vi "Internet Version Check.vi"(8 "error in":errorcluster, 9 "Prompt If Newer Version Available":bool=TRUE, 10 "Version In":dbl format="%.2f", 11 "Version File Name":string="ljstreamud.txt") -> (0 "error out":errorcluster, 1 "Newer Version Online":bool, 2 "Value (float)":dbl format="%.6f")   [LabVIEW 2021]
panel:
  out "Content":string
  out "Header":string
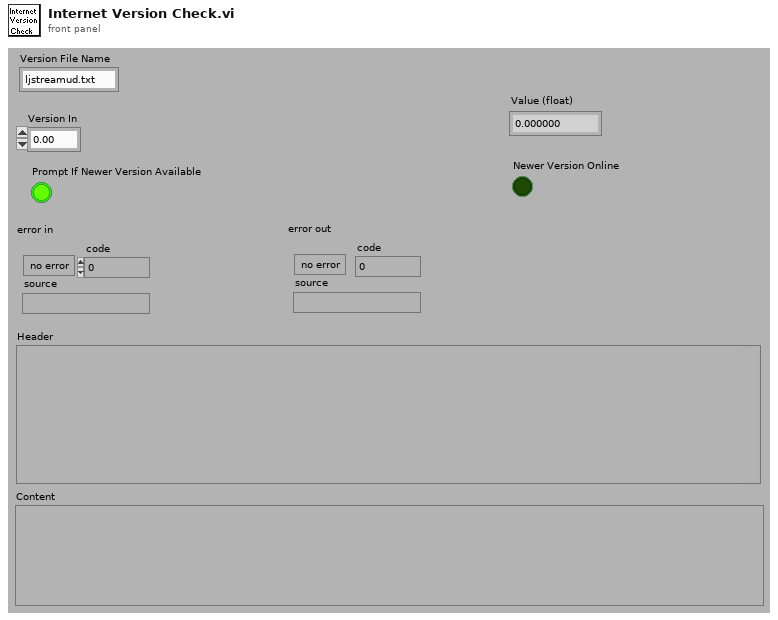
[diagram p1: front panel]
types:
  T1 = enum16{"Standard", "Buffered", "CRLF", "Immediate"}
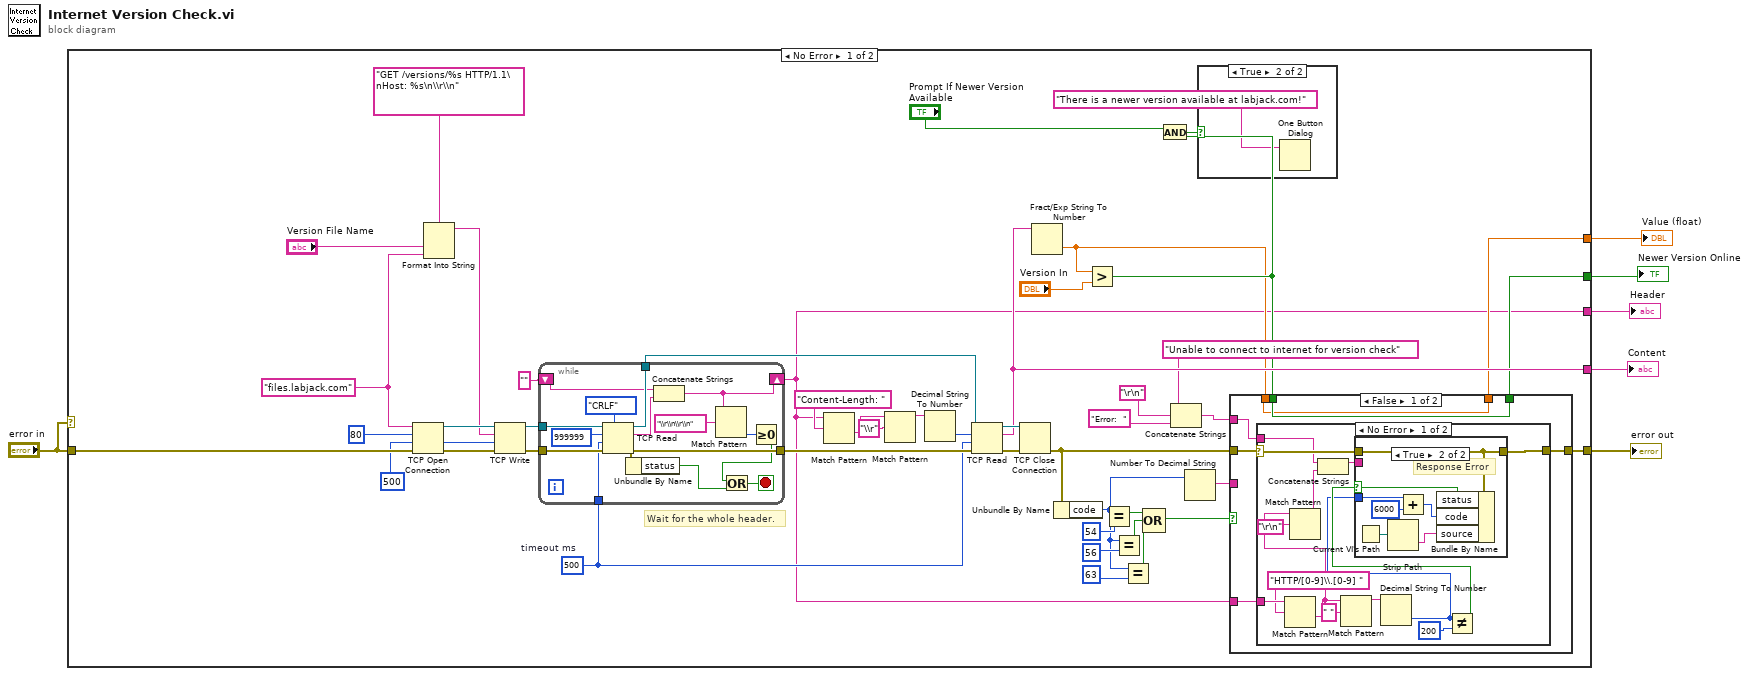
[diagram p0: block diagram]
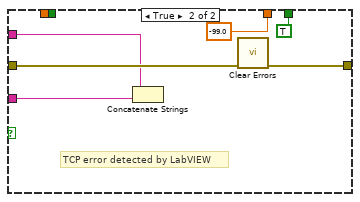
[diagram p4: hidden frame]
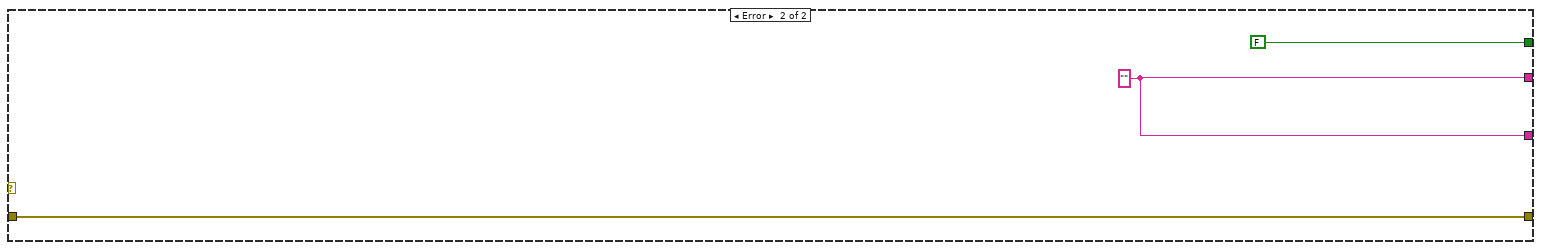
[diagram p6: hidden frame]
diagram:
  n1 = case shown="No Error" "error in" {
    tunnel: [w35 w106] -> w6
    tunnel: "error in" -> [w48 w106]
    tunnel: [w30 w105] -> w5
    tunnel: [w7 w105] -> w4
    tunnel: [w25 FALSE] -> w2
    tunnel: [w23 _] -> w1
    frame No Error {
      w22 = 500 ("timeout ms (60000)")
      w39 = 500  # timeout ms
      w32 = "files.labjack.com"
      # "Wait for the whole header."
      n2 = TCP Open Connection(address=w32, remote port or service name=u16 80 ("remote port"), timeout ms (60000)=w22, error in (no error)=w48) -> (connection ID=w52:refnum<k5>, error out=w50:errorcluster)  [unwired: 1 in]
      n3 = Format Into String(format string="GET /versions/%s HTTP/1.1\nHost: %s\n\\r\\n" ("Format String"), "Version File Name", w32) -> (resulting string=w31:string)  [unwired: 2 in, 1 out]
      n4 = TCP Write(connection ID=w52, data in=w31, error in (no error)=w50, 9:w22) -> (connection ID out=w51:refnum<k5>, error out=w49:errorcluster)  [unwired: 1 out]
      n5 = while {
        tunnel: w39 -> [w88]
        shift-left: "" -> [w98]
        shift-right: [w94] -> w7
        tunnel: [w96] -> w41
        tunnel: w49 -> [w100]
        tunnel: [w101] -> w38
        tunnel: w51 -> [w102]
        stop <- w90 stop-if-true
        n6 = TCP Read(connection ID=w102, bytes to read=999999, error in (no error)=w100, 7:T1."CRLF" ("mode (standard)"), 9:w88) -> (connection ID out=w101:refnum<k5>, data out=w97:string, error out=w96:errorcluster)
        n7 = Unbundle By Name(w96) -> ("status"=w91:bool)
        n8 = Concatenate Strings(w98, w97) -> (w94:string)
        n9 = Match Pattern(string=w94, regular expression="\\r\\n\\r\\n") -> (offset past match=w93:i32)  [unwired: 1 in, 3 out]
        n10 = Greater Or Equal To 0?(x=w93) -> (x >= 0?=w92:bool)
        n11 = Or(x=w92, y=w91) -> (x .or. y?=w90:bool)
      }
      n12 = Match Pattern(string=w7, regular expression="Content-Length: ") -> (after substring=w43:string)  [unwired: 1 in, 3 out]
      n13 = Match Pattern(string=w43, regular expression="\\r") -> (before substring=w42:string)  [unwired: 1 in, 3 out]
      n14 = Decimal String To Number(string=w42) -> (number=w40:i32)  [unwired: 2 in, 1 out]
      n15 = TCP Read(connection ID=w38, bytes to read=w40, error in (no error)=w41, 9:w39) -> (connection ID out=w37:refnum<k5>, data out=w30:string, error out=w36:errorcluster)  [unwired: 1 in]
      n16 = TCP Close Connection(connection ID=w37, error in (no error)=w36) -> (error out=w9:errorcluster)  [unwired: 1 in, 1 out]
      n17 = Fract/Exp String To Number(string=w30) -> (number=w24:dbl)  [unwired: 3 in, 1 out]
      n18 = Unbundle By Name(w9) -> ("code"=w10:i32)
      n19 = Greater?(x=w24, y="Version In") -> (0:w26:bool)
      n20 = Equal?(x=w10, y=54 ("code")) -> (x = y?=w18:bool)
      n21 = Equal?(x=w10, y=56 ("code")) -> (x = y?=w17:bool)
      n22 = Equal?(x=w10, y=63 ("code")) -> (x = y?=w16:bool)
      n23 = Compound Arithmetic op=OR(w18, w17, w16) -> (w15:bool)
      n24 = And(x="Prompt If Newer Version Available", y=w26) -> (x .and. y?=w28:bool)
      n25 = Concatenate Strings("Unable to connect to internet for version check" ("message"), "\r\n", "Error:  " ("string")) -> (w11:string)
      n26 = Number To Decimal String(number=w10) -> (decimal integer string=w8:string)  [unwired: 1 in]
      n27 = case shown="True" w28 {
        frame False {
        }
        frame True {
          n28 = One Button Dialog(message="There is a newer version available at labjack.com!") -> ()  [unwired: 1 in, 1 out]
        }
      }
      n29 = case shown="False" w15 {
        tunnel: w9 -> [w58 w86]
        tunnel: w7 -> [w57 _]
        tunnel: [w56 w87] -> w35
        tunnel: w26 -> [w55 _]
        tunnel: [w55 TRUE] -> w25
        tunnel: w24 -> [w54 _]
        tunnel: [w54 -99.0 ("Value (float)")] -> w23
        tunnel: w11 -> [w53 w83]
        tunnel: w8 -> [_ w82]
        frame False {
          n30 = case shown="No Error" w58 {
            selector: w58 -> [w68 w81]
            tunnel: [w67 w81] -> w56
            tunnel: w57 -> [w65 _]
            tunnel: w53 -> [w63 _]
            frame No Error {
              n31 = Match Pattern(string=w65, regular expression="HTTP/[0-9]\\.[0-9] ") -> (after substring=w61:string)  [unwired: 1 in, 3 out]
              n32 = Match Pattern(string=w61, regular expression="\r\n") -> (before substring=w62:string)  [unwired: 1 in, 3 out]
              n33 = Concatenate Strings(w63, w62) -> (w59:string)
              n34 = Match Pattern(string=w61, regular expression=" ") -> (before substring=w72:string)  [unwired: 1 in, 3 out]
              n35 = Decimal String To Number(string=w72) -> (number=w66:i32)  [unwired: 2 in, 1 out]
              n36 = Not Equal?(x=w66, y=200) -> (x != y?=w69:bool)
              n37 = case shown="True" w69 {
                selector: w69 -> [_ w75]
                tunnel: w68 -> [w73 w74]
                tunnel: [w73 w74] -> w67
                tunnel: w66 -> [_ w76]
                tunnel: w59 -> [_ _]
                frame False {
                }
                frame True {
                  # "Response Error"
                  n38 = Current VI's Path() -> (path=w79:path)
                  n39 = Strip Path(path=w79) -> (name=w80:string)  [unwired: 1 out]
                  n40 = Add(x=w76, y=6000) -> (x+y=w78:i32)
                  n41 = Bundle By Name(cluster=w74, "status"=w75, "code"=w78, "source"=w80) -> ()  [unwired: 1 out]
                }
              }
            }
            frame Error {
            }
          }
        }
        frame True {
          # "TCP error detected by LabVIEW"
          n42 = Concatenate Strings(w83, w82) -> ()  [unwired: 1 out]
          n43 = call <vilib>:"Clear Errors.vi"("error in (no error)"=w86) -> ("error out"=w87:errorcluster)  [unwired: 5 in, 1 out]
        }
      }
    }
    frame Error {
      w105 = ""
    }
  }
  "error out" <- w6
  "Content" <- w5
  "Header" <- w4
  "Newer Version Online" <- w2
  "Value (float)" <- w1
